vi "publish -- pll parameters.vi"(7 "publisher action":T6, 11 "pll parameters":T1={"PID parameters"={"I (sec)"=0.004634123928756344, "P (sec)"=0.008980860327047186}, "PID mode"=enum."normal", "lorentzian"={"A (VHz)"=0.0007250653088846297, "f (Hz)"=45017.43809779818, "G (Hz)"=34.46000858512321, "phi(rad)"=-1.525051560312372, "Q"=1306.3675821959234, "Norm  Ampl"=nan, "bg (V)"=7.168586400274938e-06+0.00021232547061132137i, "4corners"={"z (-pi/2)"=-1.288800856206544e-05+0.00019034453621736468i, "z(inf)"=7.168586400274938e-06+0.00021232547061132137i, "z (pi/2)"=-1.4812347993681768e-05+0.00023238206557366173i, "z center"=-1.3850178277873603e-05+0.0002113633008955132i, "z(0)"=-3.486894295602214e-05+0.00021040113117970505i, "radius"=2.1040775631078887e-05}}, "plot hist time (sec)"=1.0, "dt (sec)"=0.001, "visc hist time (sec)"=2.0, "time int ave time (sec)"=0.3, "PLL limits (Hz)"=5000.0, "PLL ON"=FALSE} {"PLL limits (Hz)" format="%#.2f"; "time int ave time (sec)" format="%#_10f"; "visc hist time (sec)" format="%#_10f"; "dt (sec)" format="%#_10f"; "plot hist time (sec)" format="%#_10f"; "lorentzian"."bg (V)" format="%#9_9f"; "lorentzian"."Q" format="%#9_9f"; "lorentzian"."phi(rad)" format="%#9_9f"; "lorentzian"."G (Hz)" format="%#9_9f"; "lorentzian"."f (Hz)" format="%#9_9f"; "PID parameters"."P (sec)" scale=0.01..10.0; "PID parameters"."I (sec)" scale=0.01..10.0}) -> (3 "pll parameters OUT":T1={"PID parameters"={"I (sec)"=0.004634123928756344, "P (sec)"=0.008980860327047186}, "PID mode"=enum."normal", "lorentzian"={"A (VHz)"=0.0007250653088846297, "f (Hz)"=45017.43809779818, "G (Hz)"=34.46000858512321, "phi(rad)"=-1.525051560312372, "Q"=1306.3675821959234, "Norm  Ampl"=nan, "bg (V)"=7.168586400274938e-06+0.00021232547061132137i, "4corners"={"z (-pi/2)"=-1.288800856206544e-05+0.00019034453621736468i, "z(inf)"=7.168586400274938e-06+0.00021232547061132137i, "z (pi/2)"=-1.4812347993681768e-05+0.00023238206557366173i, "z center"=-1.3850178277873603e-05+0.0002113633008955132i, "z(0)"=-3.486894295602214e-05+0.00021040113117970505i, "radius"=2.1040775631078887e-05}}, "plot hist time (sec)"=1.0, "dt (sec)"=0.001, "visc hist time (sec)"=2.0, "time int ave time (sec)"=0.3, "PLL limits (Hz)"=5000.0, "PLL ON"=FALSE} {"PLL limits (Hz)" format="%#.2f"; "time int ave time (sec)" format="%#_10f"; "visc hist time (sec)" format="%#_10f"; "dt (sec)" format="%#_10f"; "plot hist time (sec)" format="%#_10f"; "lorentzian"."bg (V)" format="%#9_9f"; "lorentzian"."Q" format="%#9_9f"; "lorentzian"."phi(rad)" format="%#9_9f"; "lorentzian"."G (Hz)" format="%#9_9f"; "lorentzian"."f (Hz)" format="%#9_9f"; "PID parameters"."P (sec)" scale=0.01..10.0; "PID parameters"."I (sec)" scale=0.01..10.0})   [LabVIEW 2018]
uses:
  pll parameters.ctl
  pid -- parameters.ctl
  PID - mode.ctl
  lorentzian.ctl
  circle corners.ctl
  publisher action.ctl
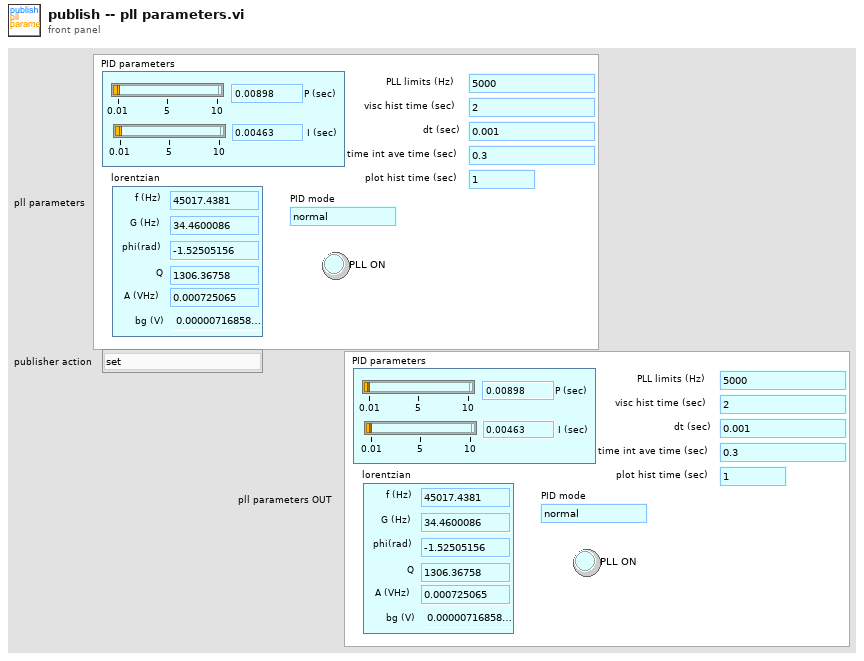
[diagram p1: front panel]
types:
  T1 = typedef "pll parameters.ctl" = cluster{"PID parameters":T2, "PID mode":T3, "lorentzian":T4, "plot hist time (sec)":dbl, "dt (sec)":dbl, "visc hist time (sec)":dbl, "time int ave time (sec)":dbl, "PLL limits (Hz)":dbl, "PLL ON":bool}
  T2 = typedef "pid -- parameters.ctl" = cluster{"I (sec)":dbl, "P (sec)":dbl}
  T3 = typedef "PID - mode.ctl" = enum16{"normal", "heat"}
  T4 = typedef "lorentzian.ctl" = cluster{"A (VHz)":dbl, "f (Hz)":dbl, "G (Hz)":dbl, "phi(rad)":dbl, "Q":dbl, "Norm  Ampl":dbl, "bg (V)":cdb, "4corners":T5}
  T5 = typedef "circle corners.ctl" = cluster{"z (-pi/2)":cdb, "z(inf)":cdb, "z (pi/2)":cdb, "z center":cdb, "z(0)":cdb, "radius":dbl}
  T6 = typedef "publisher action.ctl" = enum16{"set", "get", "init", "check"}
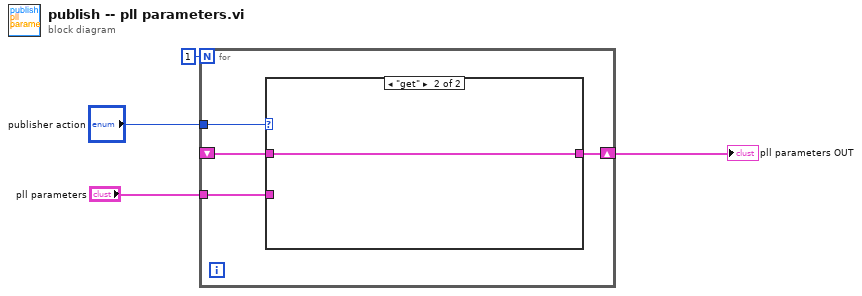
[diagram p0: block diagram]
diagram:
  n1 = for {
    N: 1 -> [_]
    tunnel: "publisher action" -> [w8]
    tunnel: "pll parameters" -> [w6]
    shift-right: [w7] -> w1
    shift-left: _ -> [w5]
    n2 = case shown="\"get\"" w8 {
      tunnel: [w9 w10] -> w7
      tunnel: w6 -> [w9 _]
      tunnel: w5 -> [_ w10]
      frame "set", Default {
      }
      frame "get" {
      }
    }
  }
  "pll parameters OUT" <- w1
